vi "DLIWebPowerSwitch.vi"(7 "Value to Output":dbl format="%.2f", 8 "Ch Description":T1={"Ch Name"="Valve8", "Type"="DLI WebPowerSwitch", "Function"=enum."Relay Output", "Ch State"=enum."On", "Calibration type"="", "A"=200.0, "B"=0.0, "C"=0.0, "D"=0.0, "Comments"="", "Address"={"Main"=0, "Ch."=1, "Sub"=0, "Port Name"="192.168.126.155"}, "String"="LV:LV", "Duty"=65535} {"Duty" format="%016b"; "D" format="%#_5g"; "C" format="%#_5g"; "B" format="%#_5g"; "A" format="%#_5g"}) -> (0 "Scan comment":string, 1 "Output":dbl format="%.3f", 3 "HelpText":string="Value to Output: >0- On, else Off\n\"Port Name\" contains the IP address of the unit\nCh. is used to specify the outlet number, 1-8\nComments (the red box) is used for username:password")   [LabVIEW 2021]
uses:
  ADAM Client/Sub VIs/ADAM Controls/Ch_description_ADAM.ctl
  ADAM Client/Sub VIs/ADAM Controls/Module_type_ADAM.ctl
  ADAM Client/Sub VIs/ADAM Controls/Function_ADAM.ctl
  ADAM Client/Sub VIs/ADAM Controls/Channel_State.ctl
  ADAM Client/Sub VIs/ADAM Controls/Calib_type_ADAM.ctl
  ADAM Client/Sub VIs/ADAM Controls/Address.ctl
  <vilib>/Utility/error.llb/DialogType.ctl
  <vilib>/httpClient/LabVIEWHTTPClient.lvlib
panel:
  out "nCalls":dbl
  out "execTime 2":dbl caption="Avg Execution Time" format="%_3ps"
  out "execTime":dbl caption="Execution Time" format="%_3ps"
  out "body":string
  out "headers":string
  # "VI to control the Digital Loggers International Web Power Switch"
  # "https://www.digital-loggers.com/lpc.html"
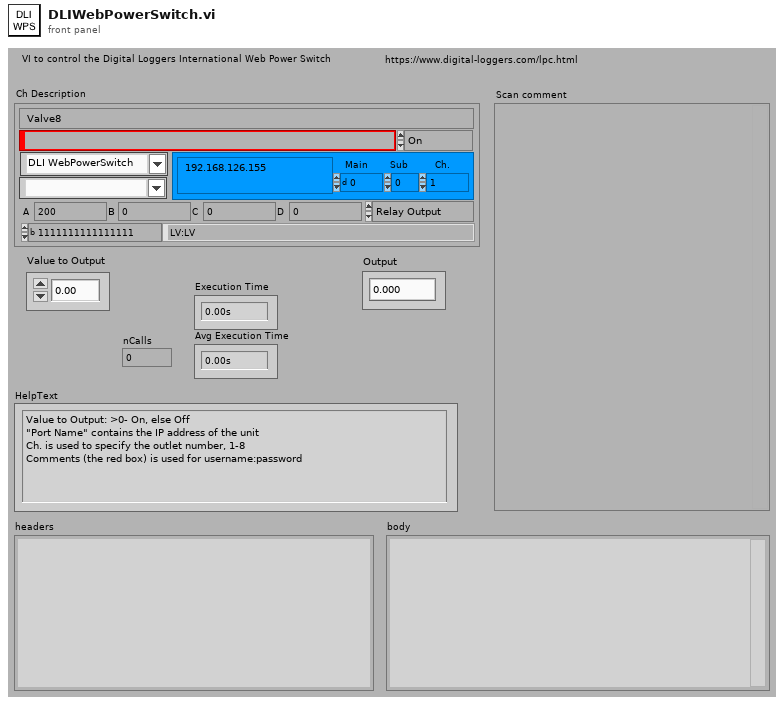
[diagram p1: front panel]
types:
  T1 = typedef "Ch_description_ADAM.ctl" = cluster{"Ch Name":string, "Type":T2, "Function":T3, "Ch State":T4, "Calibration type":T5, "A":dbl, "B":dbl, "C":dbl, "D":dbl, "Comments":string, "Address":T6, "String":string, "Duty":u16}
  T2 = typedef "Module_type_ADAM.ctl" = string
  T3 = typedef "Function_ADAM.ctl" = enum16{"Analogue Input", "Digital Input", "Event counter", "Event rate", "Analogue Output", "Digital Output", "Relay Output"}
  T4 = typedef "Channel_State.ctl" = enum16{"On", "Off", "Always On", "Always Off"}
  T5 = typedef "Calib_type_ADAM.ctl" = string
  T6 = typedef "Address.ctl" = cluster{"Main":i32, "Ch.":i32, "Sub":i32, "Port Name":string}
  T7 = typedef "DialogType.ctl" = u16
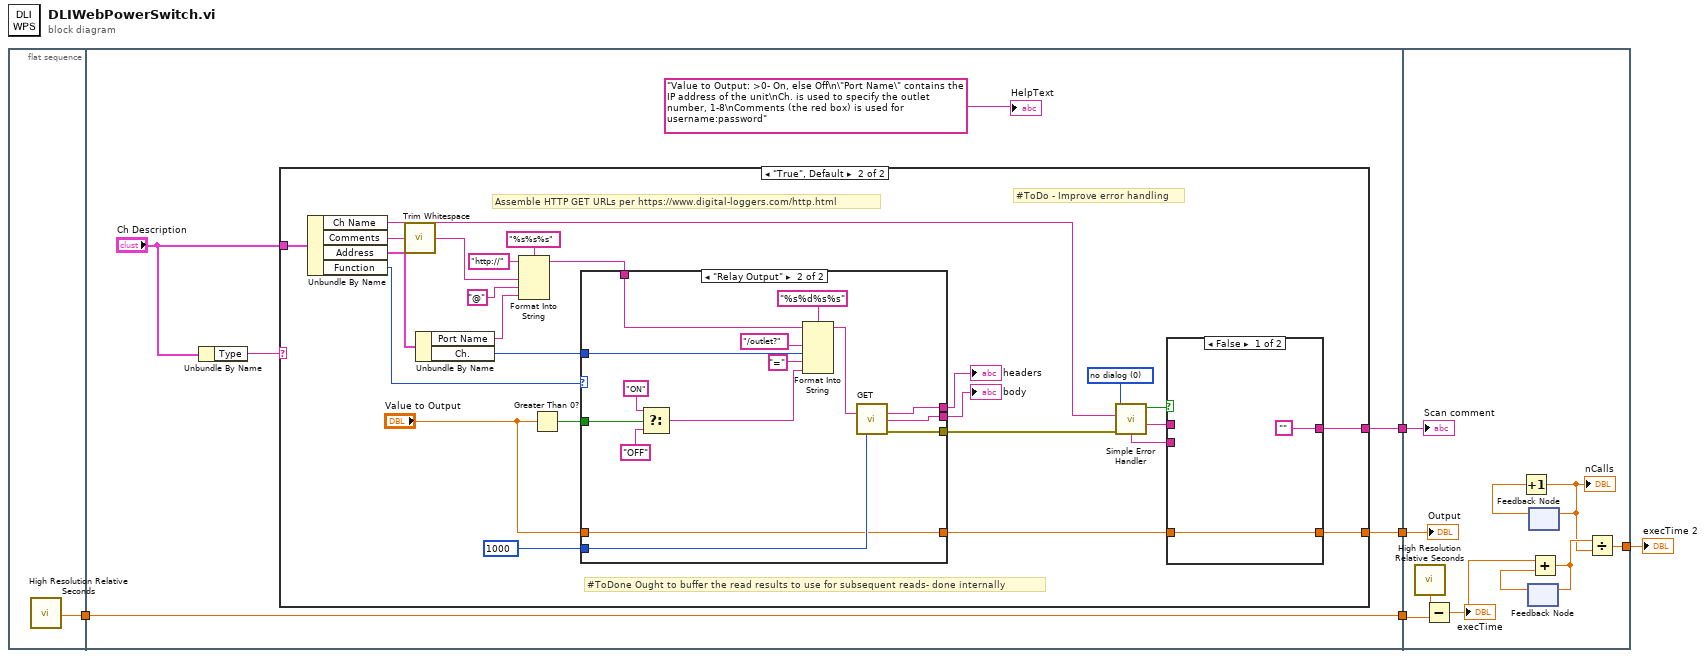
[diagram p0: block diagram]
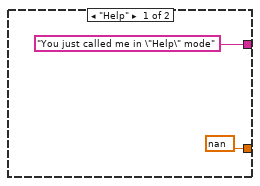
[diagram p2: hidden frame]
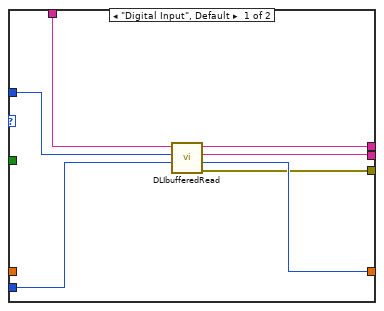
[diagram p3: hidden frame]
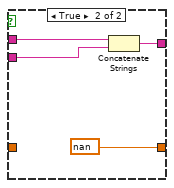
[diagram p4: hidden frame]
diagram:
  n1 = flat-sequence {
    tunnel: [w6] -> w3
    tunnel: [w9] -> w5
    tunnel: [w8] -> w4
    tunnel: w3 -> [w7]
    tunnel: [w7] -> w2
    tunnel: w5 -> [w77]
    tunnel: w4 -> [w76]
    tunnel: w2 -> [w74]
    tunnel: [w68] -> w1
    frame #0 {
      n2 = call <vilib>:"High Resolution Relative Seconds.vi"() -> ("relative seconds"=w6:dbl)
    }
    frame #1 {
      n3 = Unbundle By Name("Ch Description") -> ("Type"=w11:T2)
      n4 = case shown="\"True\", Default" w11 {
        tunnel: ["You just called me in \"Help\" mode" w34] -> w9
        tunnel: [nan ("t") w33] -> w8
        tunnel: "Ch Description" -> [_ w25]
        frame "Help" {
        }
        frame "True", Default {
          w39 = T7 0 items=["no dialog", "OK message", "continue or stop message", "OK message + warnings", "continue/stop + warnings"] ("type of dialog (OK msg:1)")
          # "#ToDone Ought to buffer the read results to use for subsequent reads- done internally"
          # "#ToDo - Improve error handling"
          # "Assemble HTTP GET URLs per https://www.digital-loggers.com/http.html"
          n5 = Unbundle By Name(w25) -> ("Ch Name"=w26:string, "Comments"=w19:string, "Address"=w36:T6, "Function"=w22:T3)
          n6 = call <vilib>:"Trim Whitespace.vi"("string"=w19) -> ("trimmed string"=w18:string)  [unwired: 1 in]
          n7 = Unbundle By Name(w36) -> ("Port Name"=w30:string, "Ch."=w27:i32)
          n8 = Format Into String(format string="%s%s%s", initial string="http://", w18, "@" ("input 2"), w30) -> (resulting string=w28:string)  [unwired: 1 in, 1 out]
          n9 = Greater Than 0?(x="Value to Output") -> (x > 0?=w17:bool)
          n10 = case shown="\"Relay Output\"" w22 {
            tunnel: [w40 w57] -> w21
            tunnel: w28 -> [w46 w56]
            tunnel: w27 -> [w45 w55]
            tunnel: 1000 ("A") -> [w44 w52]
            tunnel: [w43 w54] -> w24
            tunnel: [w42 w53] -> w23
            tunnel: [w41 w47] -> w20
            tunnel: w17 -> [_ w48]
            tunnel: "Value to Output" -> [_ w47]
            frame "Digital Input", Default {
              n11 = call "DLIbufferedRead.vi"("timeout(ms)"=w44, "Ch."=w45, "URL"=w46) -> ("error out"=w40:errorcluster, "state(1or0)"=w41:i16, "body"=w42:string, "headers"=w43:string)  [unwired: 5 in]
            }
            frame "Relay Output" {
              n12 = Select(t="ON", s=w48, f="OFF") -> (s? t:f=w49:string)
              n13 = Format Into String(format string="%s%d%s%s", initial string=w56, "/outlet?" ("input 4"), w55, "=", w49) -> (resulting string=w58:string)  [unwired: 1 in, 1 out]
              n14 = call <vilib>:"GET.vi"("url"=w58, "timeout (10000)"=w52) -> ("headers"=w54:string, "body"=w53:string, "error out"=w57:errorcluster)  [unwired: 10 in, 1 out]
            }
          }
          "headers" <- w24
          "body" <- w23
          n15 = call <vilib>:"Simple Error Handler.vi"("error source (\" \")"=w26, "type of dialog (OK msg:1)"=w39, "error in (no error)"=w21) -> ("error?"=w35:bool, "source out"=w37:string, "message"=w38:string)  [unwired: 4 out]
          n16 = case shown="False" w35 {
            tunnel: w38 -> [_ w65]
            tunnel: w37 -> [_ w66]
            tunnel: ["" w64] -> w34
            tunnel: [w62 nan ("t")] -> w33
            tunnel: w20 -> [w62 _]
            frame False {
            }
            frame True {
              n17 = Concatenate Strings(w66, w65) -> (w64:string)
            }
          }
        }
      }
      "HelpText" <- "Value to Output: >0- On, else Off\n\"Port Name\" contains the IP address of the unit\nCh. is used to specify the outlet number, 1-8\nComments (the red box) is used for username:password"
    }
    frame #2 {
      n18 = call <vilib>:"High Resolution Relative Seconds.vi"() -> ("relative seconds"=w75:dbl)
      n19 = Subtract(x=w75, y=w74) -> (x-y=w73:dbl)
      "execTime" <- w73
      n20 = feedback #1() -> (w72:dbl)  [unwired: 1 in]
      n21 = feedback #2() -> (w71:dbl)  [unwired: 1 in]
      n22 = Increment(x=w71) -> (x+1=w69:dbl)
      "nCalls" <- w69
      n23 = feedback-in #2(w69) -> ()
      n24 = Add(x=w73, y=w72) -> (x+y=w70:dbl)
      n25 = feedback-in #1(w70) -> ()
      n26 = Divide(x=w70, y=w69) -> (x/y=w68:dbl)
      "Scan comment" <- w77
      "Output" <- w76
    }
  }
  "execTime 2" <- w1
